vi "CLAElevatorMain.vi"() -> ()   [LabVIEW 2020]
uses:
  Support/ErrorHandler/ErrorHandler.lvlib
  Controller/Controller.lvlib
  Support/UserEvents/Controls/EventMessage.ctl
  SensorInterface/SensorInterface.lvlib
panel:
  out "error out":errorcluster
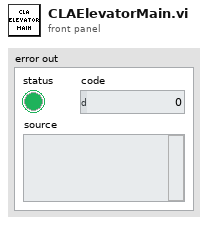
[diagram p1: front panel]
types:
  T1 = typedef "EventMessage.ctl" = cluster{"Command":string, "Data":variant}
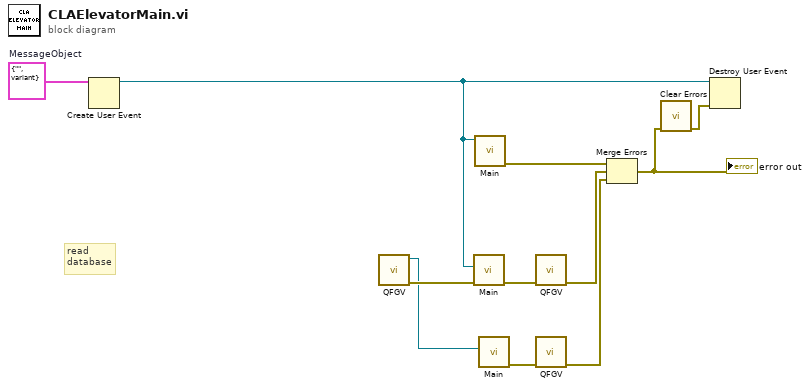
[diagram p0: block diagram]
diagram:
  w8 = T1 {"Command"="", "Data"=variant}  # MessageObject
  # "read \ndatabase"
  n1 = Create User Event(user event datatype=w8) -> (user event=w1:refnum<user-event>)  [unwired: 1 in, 1 out]
  n2 = call "QFGV.vi"() -> ("error out"=w11:errorcluster, "ModuleQ"=w3:refnum<queue>)  [unwired: 10 in]
  n3 = call "Main.vi"("error in (no error)"=w11, "UIEvents"=w1) -> ("error out"=w9:errorcluster)  [unwired: 8 in, 1 out]
  n4 = call "Main.vi"("UIEvents"=w1) -> ("error out"=w2:errorcluster)  [unwired: 10 in]
  n5 = call "Main.vi"("ControllerQ"=w3) -> ("error out"=w10:errorcluster)  [unwired: 9 in, 1 out]
  n6 = call "QFGV.vi"("error in (no error)"=w9) -> ("error out"=w6:errorcluster)  [unwired: 9 in, 1 out]
  n7 = call "QFGV.vi"("error in (no error)"=w10) -> ("error out"=w7:errorcluster)  [unwired: 9 in, 1 out]
  n8 = Merge Errors(w2, w6, w7) -> (w5:errorcluster)
  "error out" <- w5
  n9 = call <vilib>:"Clear Errors.vi"("error in (no error)"=w5) -> ("error out"=w4:errorcluster)  [unwired: 5 in, 1 out]
  n10 = Destroy User Event(user event=w1, error in=w4) -> ()  [unwired: 1 out]
